vi "Initiate Upload.vi"(8 "Error In":errorcluster, 10 "Number of Waypoints":u16=6, 11 "Aircraft Index":u8) -> (0 "Error Out":errorcluster)   [LabVIEW 2014]
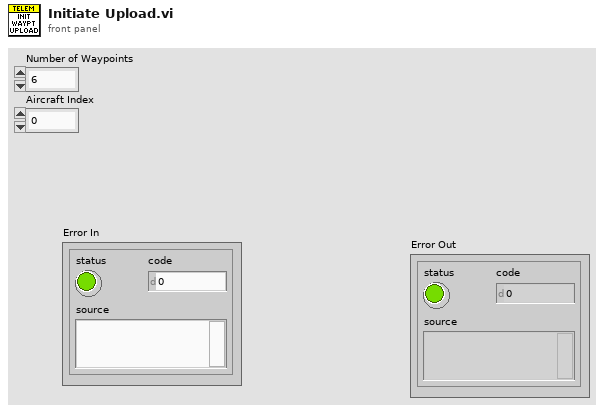
[diagram p1: front panel]
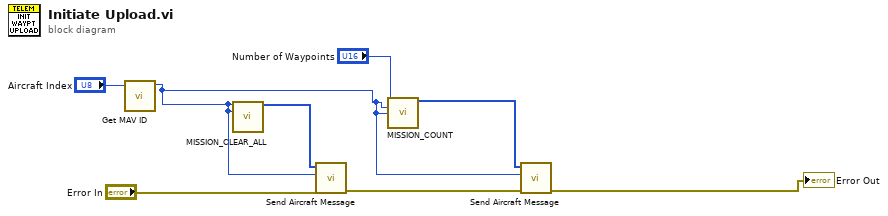
[diagram p0: block diagram]
diagram:
  n1 = call "Get MAV ID.vi"("Aircraft Index"="Aircraft Index") -> ("Aircraft ID"=w2:u8)  [unwired: 9 in, 1 out]
  n2 = call "MISSION_CLEAR_ALL.vi"("target_system"=w2, "target_component"=w2) -> ("MAVLink Message"=w5:u8[])  [unwired: 13 in]
  n3 = call "Send Aircraft Message.vi"("error in (no error)"="Error In", "Aircraft ID"=w2, "MAVLink Message"=w5) -> ("error out"=w4:errorcluster)  [unwired: 8 in]
  n4 = call "MISSION_COUNT.vi"("count"="Number of Waypoints", "target_system"=w2, "target_component"=w2) -> ("MAVLink Message"=w3:u8[])  [unwired: 12 in]
  n5 = call "Send Aircraft Message.vi"("error in (no error)"=w4, "Aircraft ID"=w2, "MAVLink Message"=w3) -> ("error out"=→"Error Out":errorcluster)  [unwired: 8 in]
